vi "Messaging Init.vi"(8 "error in (no error)":errorcluster, 11 "References Name (in)":string) -> (0 "error out":errorcluster, 2 "References Name (out)":string, 3 "Messaging out":refnum<class "Messaging.lvclass">)   [LabVIEW 2023, in "Messaging.lvclass"]
doc: "This method serves as a constructor for the Messaging Class. Use this to instantiate a class."
uses:
  Messaging.lvclass
  Messaging.lvclass/Messaging.ctl
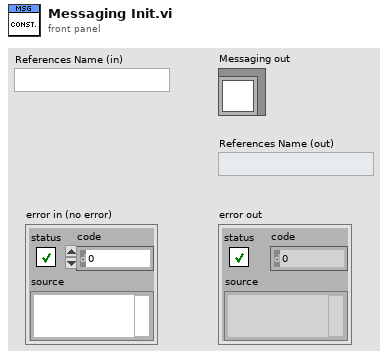
[diagram p1: front panel]
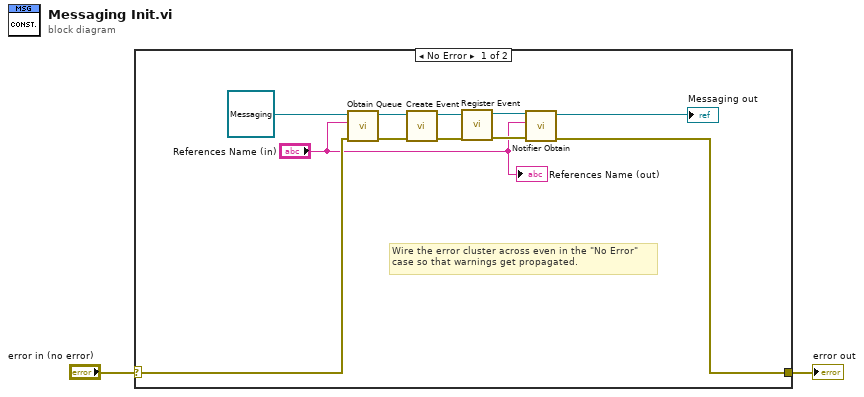
[diagram p0: block diagram]
diagram:
  n1 = case shown="No Error" "error in (no error)" {
    selector: "error in (no error)" -> [w8 w14]
    tunnel: [w5 w14] -> w1
    frame No Error {
      # "Wire the error cluster across even in the \"No Error\"\ncase so that warnings get propagated."
      n2 = call "Obtain Queue.vi"("error in (no error)"=w8, "Queue Name (in)"="References Name (in)", "Messaging in"=refnum<class "Messaging.lvclass"> refnum ("Messaging.lvclass")) -> ("error out"=w12:errorcluster, "Messaging out"=w11:refnum<class "Messaging.lvclass">)  [unwired: 7 in]
      n3 = call "Create Event.vi"("error in (no error)"=w12, "Messaging in"=w11) -> ("error out"=w9:errorcluster, "Messaging out"=w10:refnum<class "Messaging.lvclass">)  [unwired: 8 in]
      n4 = call "Register Event.vi"("error in (no error)"=w9, "Messaging in"=w10) -> ("error out"=w6:errorcluster, "Messaging out"=w7:refnum<class "Messaging.lvclass">)  [unwired: 8 in]
      n5 = call "Notifier Obtain.vi"("error in (no error)"=w6, "Notifier Name"="References Name (in)", "Messaging in"=w7) -> ("error out"=w5:errorcluster, "Messaging out"=→"Messaging out":refnum<class "Messaging.lvclass">)  [unwired: 7 in]
      "References Name (out)" <- "References Name (in)"
    }
    frame Error {
    }
  }
  "error out" <- w1
